vi "Point-in-Box test (axis-aligned).vi"(1 "Point":sgl[](array[numeric]), 2 "Box":T1) -> (0 "Point is inside box":bool)   [LabVIEW 2014]
uses:
  Typedefs/TreeNodeBox.ctl
  Typedefs/Quad.ctl
  Typedefs/Quadplane enum.ctl
panel:
  # "PN 17/01/2015"
  # "Vertices"
  # "Edges"
  # "Unit normal"
  # "Plane ident."
  # "Vertices"
  # "Edges"
  # "Unit normal"
  # "Plane ident."
  # "Vertices"
  # "Edges"
  # "Unit normal"
  # "Plane ident."
  # "Vertices"
  # "Edges"
  # "Unit normal"
  # "Plane ident."
  # "Vertices"
  # "Edges"
  # "Unit normal"
  # "Plane ident."
  # "Vertices"
  # "Edges"
  # "Unit normal"
  # "Plane ident."
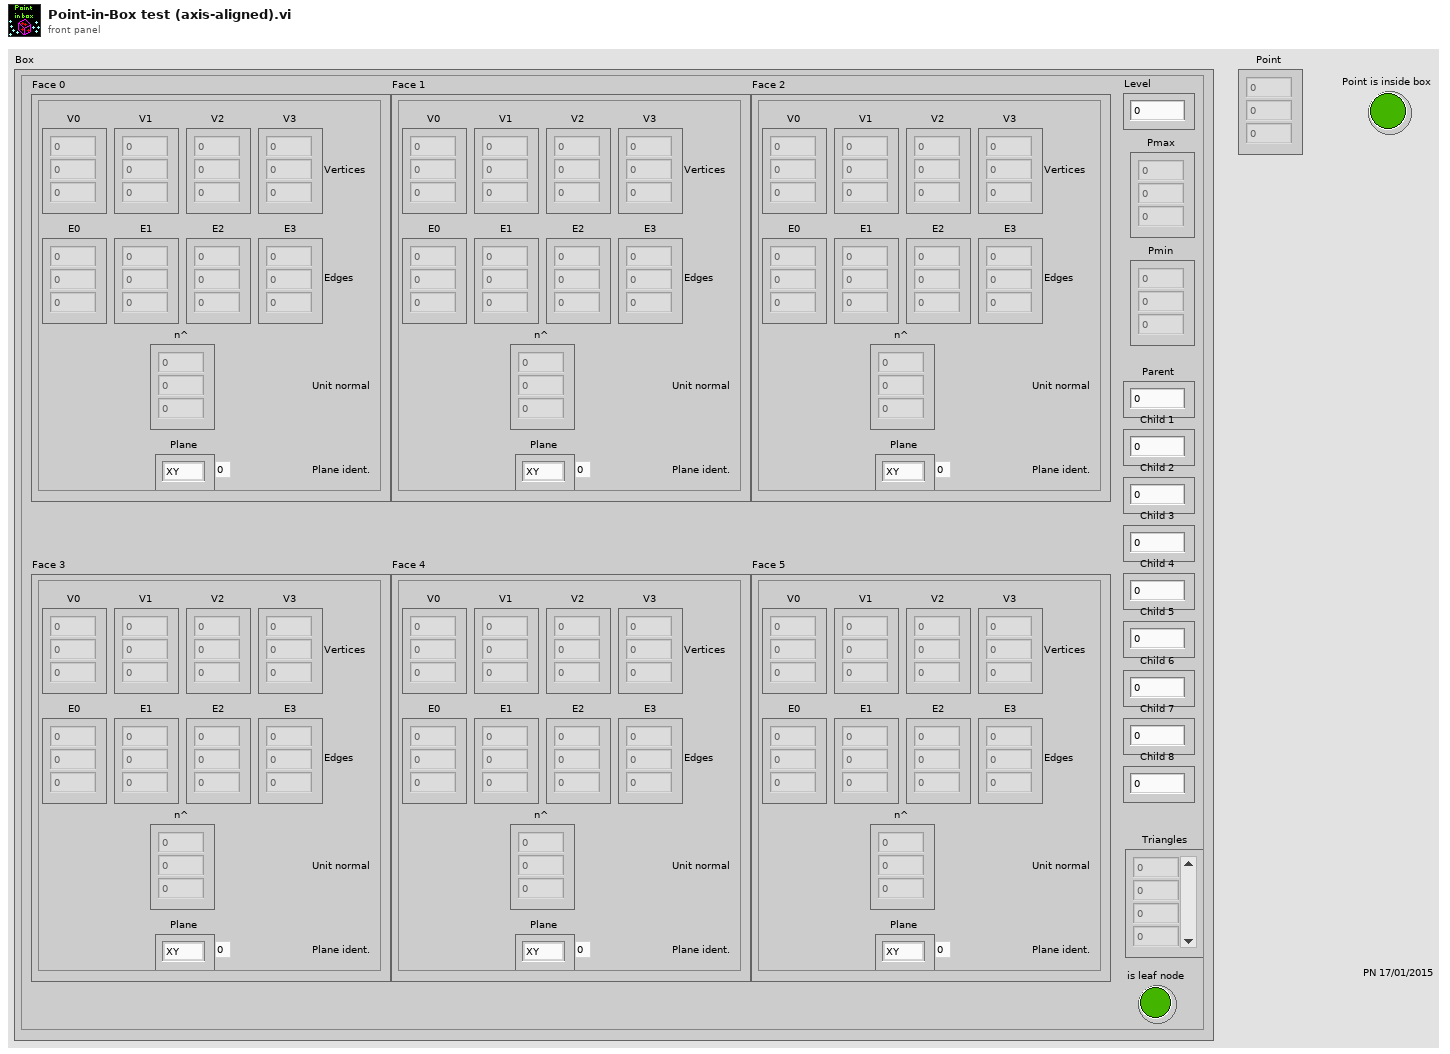
[diagram p1: front panel]
types:
  T1 = typedef "TreeNodeBox.ctl" = cluster{"Face 0":T2, "Face 1":T2, "Face 2":T2, "Face 3":T2, "Face 4":T2, "Face 5":T2, "Level":i32, "Pmax":sgl[], "Pmin":sgl[], "Parent":i32, "Child 1":i32, "Child 2":i32, "Child 3":i32, "Child 4":i32, "Child 5":i32, "Child 6":i32, "Child 7":i32, "Child 8":i32, "Triangles":i32[], "is leaf node":bool}
  T2 = typedef "Quad.ctl" = cluster{"V0":sgl[], "V1":sgl[], "V2":sgl[], "V3":sgl[], "E0":sgl[], "E1":sgl[], "E2":sgl[], "E3":sgl[], "n^":sgl[], "Plane":T3}
  T3 = typedef "Quadplane enum.ctl" = enum8{"XY", "XZ", "YZ", "-XY", "-XZ", "-YZ"}
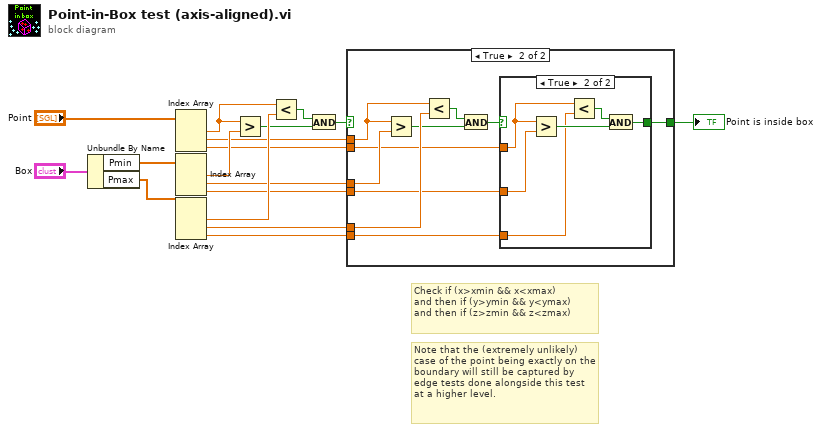
[diagram p0: block diagram]
diagram:
  # "Note that the (extremely unlikely) case of the point being exactly on the boundary will still be captured by edge tests done alongside this test at a higher level."
  # "Check if (x>xmin && x<xmax)\nand then if (y>ymin && y<ymax)\nand then if (z>zmin && z<zmax)"
  n1 = Unbundle By Name("Box") -> ("Pmin"=w15:sgl[], "Pmax"=w14:sgl[])
  n2 = Index Array(array="Point") -> (element #1=w11:sgl, element #2=w6:sgl, element #3=w1:sgl)  [unwired: 3 in]
  n3 = Index Array(array=w15) -> (element #1=w12:sgl, element #2=w5:sgl, element #3=w2:sgl)  [unwired: 3 in]
  n4 = Index Array(array=w14) -> (element #1=w10:sgl, element #2=w4:sgl, element #3=w3:sgl)  [unwired: 3 in]
  n5 = Greater?(x=w11, y=w12) -> (0:w8:bool)
  n6 = Less?(x=w11, y=w10) -> (x < y?=w9:bool)
  n7 = And(x=w9, y=w8) -> (x .and. y?=w7:bool)
  n8 = case shown="True" w7 {
    selector: w7 -> [w18 _]
    tunnel: w6 -> [_ w27]
    tunnel: w5 -> [_ w28]
    tunnel: w4 -> [_ w26]
    tunnel: w3 -> [_ w22]
    tunnel: w2 -> [_ w21]
    tunnel: w1 -> [_ w20]
    tunnel: [w18 w19] -> w13
    frame False {
    }
    frame True {
      n9 = Greater?(x=w27, y=w28) -> (0:w24:bool)
      n10 = Less?(x=w27, y=w26) -> (x < y?=w25:bool)
      n11 = And(x=w25, y=w24) -> (x .and. y?=w23:bool)
      n12 = case shown="True" w23 {
        selector: w23 -> [w29 _]
        tunnel: w22 -> [_ w33]
        tunnel: w21 -> [_ w32]
        tunnel: w20 -> [_ w31]
        tunnel: [w29 w30] -> w19
        frame False {
        }
        frame True {
          n13 = Greater?(x=w31, y=w32) -> (0:w35:bool)
          n14 = Less?(x=w31, y=w33) -> (x < y?=w34:bool)
          n15 = And(x=w34, y=w35) -> (x .and. y?=w30:bool)
        }
      }
    }
  }
  "Point is inside box" <- w13
